vi "ini_load.vi"(8 "error in":errorcluster, 11 "items command":string) -> (0 "error out":errorcluster)   [LabVIEW 2020]
uses:
  <vilib>/Utility/config.llb/NI_LVConfig.lvlib
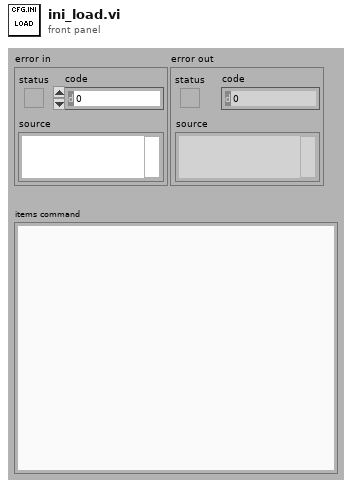
[diagram p1: front panel]
types:
  T1 = typedef "NI_LVConfig.lvlib/Config Data RefNum.ctl" = refnum<k1>
  T2 = typedef "ini_parse_row.ctl" = cluster{"ini section":string, "ini key":string, "ini default":string, "control ref":refnum<vi>, "uid":i32, "vi ref":refnum<vi>}
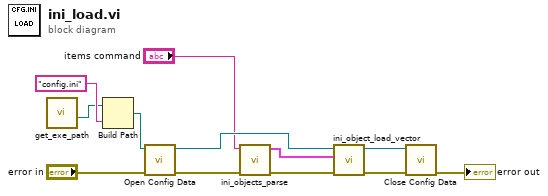
[diagram p0: block diagram]
diagram:
  n1 = call "get_exe_path.vi"() -> ("directory path"=w1:path)  [unwired: 3 out]
  n2 = Build Path(base path=w1, name or relative path="config.ini") -> (appended path=w10:path)
  n3 = call <vilib>:"Open Config Data.vi"("error in (no error)"="error in", "configuration file path"=w10) -> ("error out"=w9:errorcluster, "refnum"=w7:T1)  [unwired: 7 in, 1 out]
  n4 = call "ini_objects_parse.vi"("error in"=w9, "items command"="items command") -> ("error out"=w8:errorcluster, "ini items"=w2:T2[])  [unwired: 8 in]
  n5 = call "ini_object_load_vector.vi"("error in"=w8, "objects to save"=w2, "refnum in"=w7) -> ("error out"=w5:errorcluster, "refnum out"=w4:T1)  [unwired: 7 in]
  n6 = call <vilib>:"Close Config Data.vi"("error in (no error)"=w5, "refnum"=w4) -> ("error out"=→"error out":errorcluster)  [unwired: 8 in, 1 out]
